vi "List Mode - Configure Sequence.vi"   [LabVIEW 2014, in "Associated Power Technologies 8500 Series.lvlib"]
uses:
  <instrlib>/Associated Power Technologies 8500 Series/Associated Power Technologies 8500 Series.lvlib
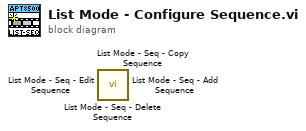
[diagram p0: block diagram]
diagram:
  n1 = call <instrlib>:"List Mode - Seq - Delete Sequence.vi"() -> ()  [unwired: 10 in, 2 out]
  n2 = call <instrlib>:"List Mode - Seq - Copy Sequence.vi"() -> ()  [unwired: 10 in, 2 out]
  n3 = call <instrlib>:"List Mode - Seq - Edit Sequence.vi"() -> ()  [unwired: 10 in, 2 out]
  n4 = call <instrlib>:"List Mode - Seq - Add Sequence.vi"() -> ()  [unwired: 10 in, 2 out]
